vi "Build All.vi"() -> ()   [LabVIEW 2021]
uses:
  <vilib>/CIF Foundation/CIF LabVIEW Scripting/LV Scripting/Typedef/Version Increment.ctl
  <vilib>/CIF Foundation/CIF LabVIEW Scripting/LV Scripting/LV Scripting Utilities.lvlib
  <vilib>/AppBuilder/AB_API_Simple/NI_App_Builder_API.lvlib
  <vilib>/AppBuilder/AB_API_Simple/Build (path).vi
panel:
  in  "String":string
  in  "Changes":string
  in  "Version Increment":T1
  out "error out":errorcluster
  out "Description":string
  out "Version":T2
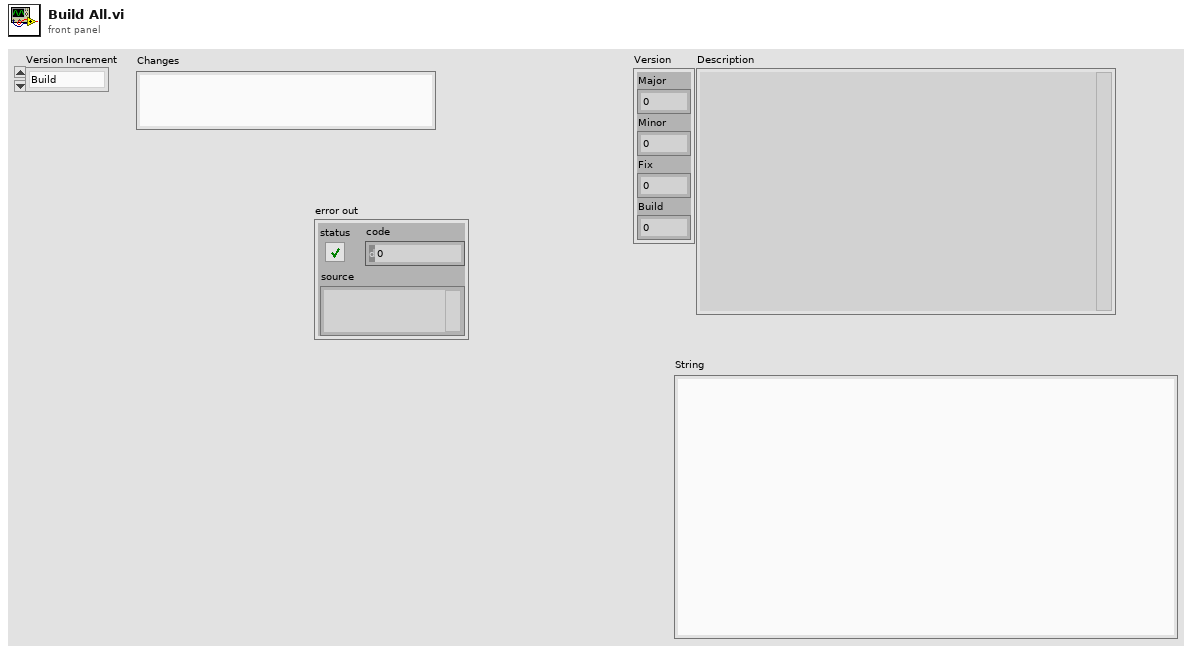
[diagram p1: front panel]
types:
  T1 = typedef "LV Scripting Utilities.lvlib/Version Increment.ctl" = enum16{"Build", "Fix", "Minor", "Major"}
  T2 = cluster{"Major":u16, "Minor":u16, "Fix":u16, "Build":u16}
  T3 = typedef "LV Scripting Utilities.lvlib/Target References.ctl" = cluster{"Target Reference":refnum<vi>, "VI References":refnum<vi>[], "Library References":refnum<vi>[], "Build References":refnum<vi>[]}
  T4 = typedef "LV Scripting Utilities.lvlib/BuildSpec Map.ctl" = map{string, refnum<vi>}
  T5 = typedef "LV Scripting Utilities.lvlib/Library Map.ctl" = map{string, refnum<vi>}
  T6 = typedef "Version.ctl" = cluster{"Major":u16, "Minor":u16, "Fix":u16, "Build":u16}
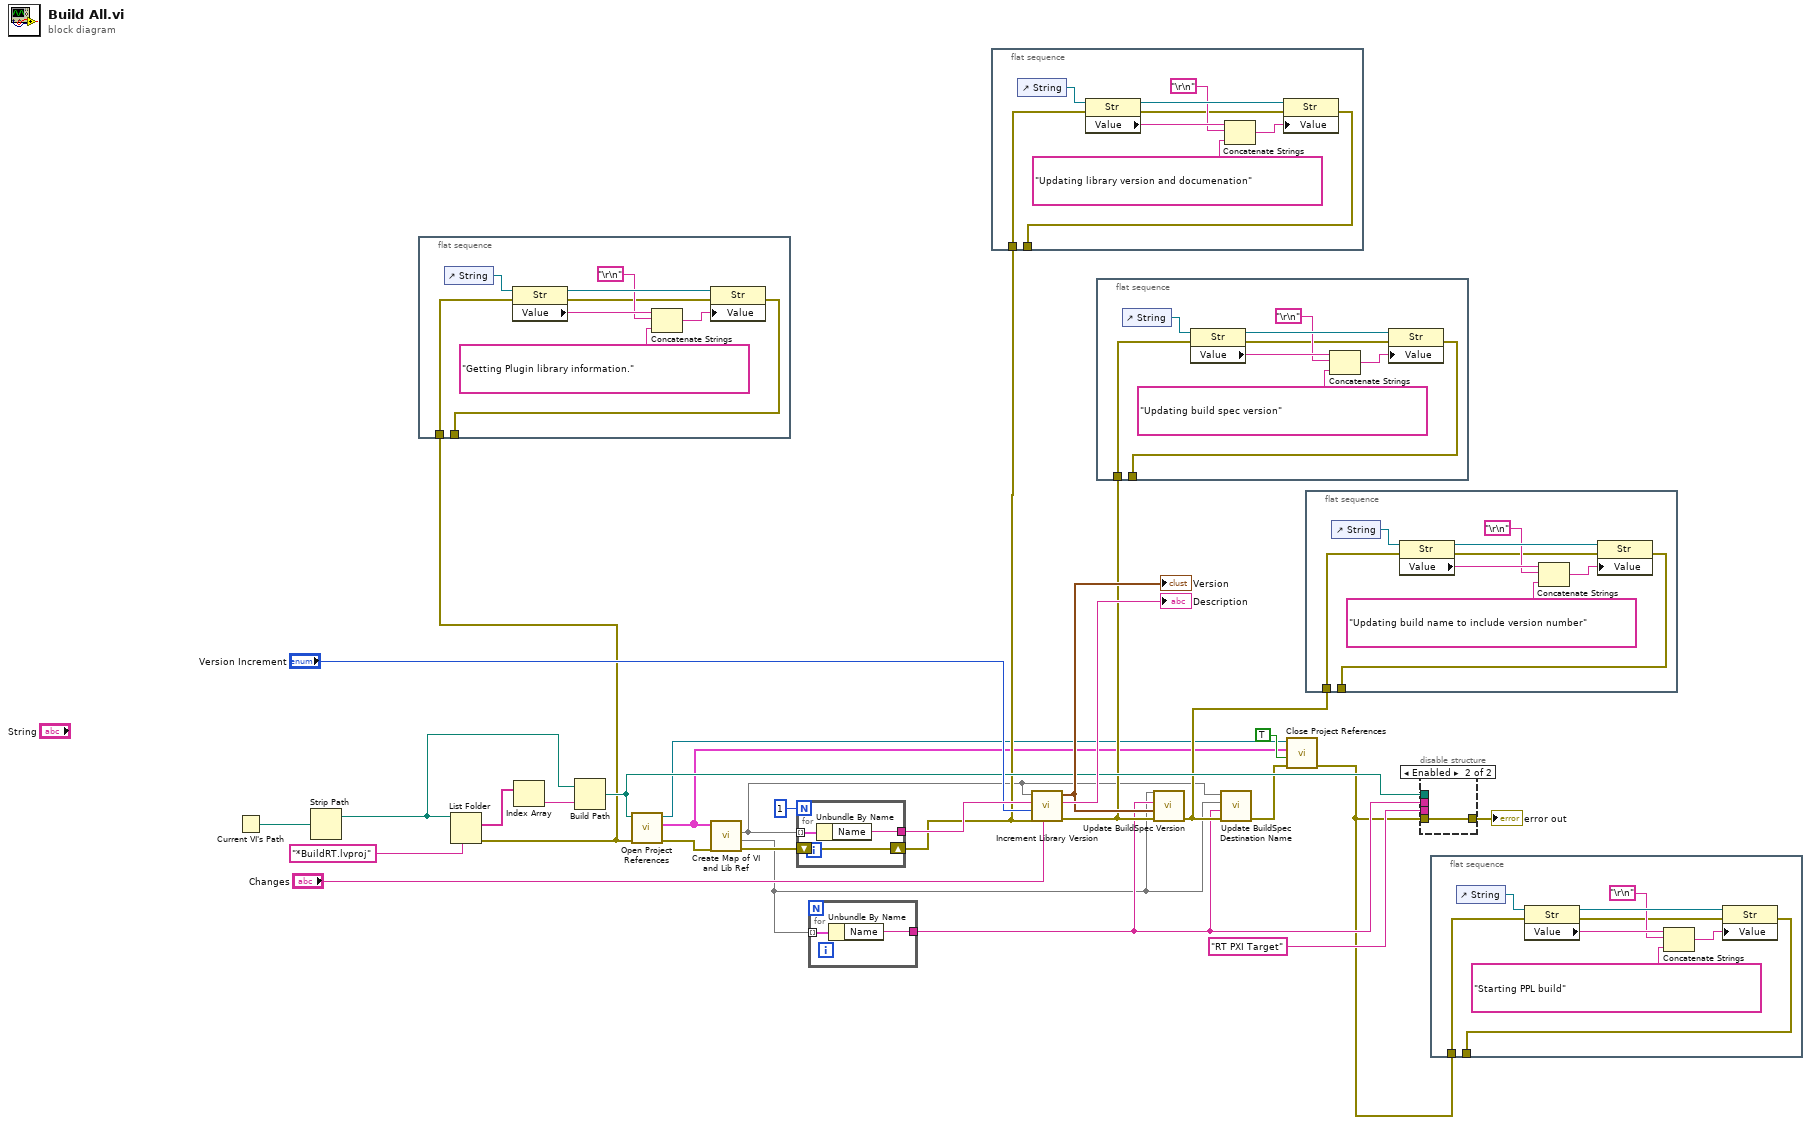
[diagram p0: block diagram]
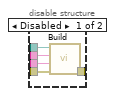
[diagram p2: hidden frame]
diagram:
  n1 = Current VI's Path() -> (path=w28:path)
  n2 = Strip Path(path=w28) -> (stripped path=w22:path)  [unwired: 1 out]
  n3 = flat-sequence {
    tunnel: w12 -> [w31]
    tunnel: [w29] -> _
    frame #0 {
      n4 = control-ref of="String"() -> (w37:refnum<vi>)
      n5 = property class="Str"(reference=w37, error in=w31) -> (reference out=w33:refnum<vi>, error out=w30:errorcluster, "Value"=w36:string)
      n6 = Concatenate Strings(w36, "\r\n", "Getting Plugin library information." ("Value")) -> (w34:string)
      n7 = property class="Str"(reference=w33, error in=w30, "Value"=w34) -> (error out=w29:errorcluster)  [unwired: 1 out]
    }
  }
  n8 = List Folder(path=w22, pattern="*BuildRT.lvproj") -> (filenames=w26:string[], error out=w12:errorcluster)  [unwired: 2 in, 2 out]
  n9 = Index Array(array=w26) -> (element=w23:string)  [unwired: 1 in]
  n10 = Build Path(base path=w22, name or relative path=w23) -> (appended path=w14:path)
  n11 = call <vilib>:"Open Project References.vi"("error in"=w12, "Project Path"=w14) -> ("error out"=w25:errorcluster, "VI, Library, and Build References"=w4:T3[], "Project Reference"=w5:refnum<vi>)  [unwired: 7 in]
  n12 = call <vilib>:"Create Map of VI and Lib Ref.vi"("error in"=w25, "VI, Library, and Build References"=w4) -> ("error out"=w20:errorcluster, "BuildSpec Map"=w7:T4, "Library Map"=w6:T5)  [unwired: 6 in, 1 out]
  n13 = for {
    N: 1 -> [_]
    tunnel: w6 -> [w40] mode=indexing
    tunnel: [w39] -> w19
    shift-right: [w38] -> w8
    shift-left: w20 -> [w38]
    n14 = Unbundle By Name(w40) -> ("Name"=w39:string)
  }
  n15 = for {
    tunnel: w7 -> [w42] mode=indexing
    tunnel: [w41] -> w9
    n16 = Unbundle By Name(w42) -> ("Name"=w41:string)
  }
  n17 = flat-sequence {
    tunnel: w8 -> [w45]
    tunnel: [w43] -> _
    frame #0 {
      n18 = control-ref of="String"() -> (w51:refnum<vi>)
      n19 = property class="Str"(reference=w51, error in=w45) -> (reference out=w47:refnum<vi>, error out=w44:errorcluster, "Value"=w50:string)
      n20 = Concatenate Strings(w50, "\r\n", "Updating library version and documenation" ("Value")) -> (w48:string)
      n21 = property class="Str"(reference=w47, error in=w44, "Value"=w48) -> (error out=w43:errorcluster)  [unwired: 1 out]
    }
  }
  n22 = call <vilib>:"Increment Library Version.vi"("Changes"="Changes", "error in (no error)"=w8, "Version Increment"="Version Increment", "Library Name"=w19, "Library Map"=w6) -> ("error out"=w11:errorcluster, "Description"=→"Description":string, "Version"=w15:T6)  [unwired: 4 in]
  "Version" <- w15
  n23 = flat-sequence {
    tunnel: w11 -> [w54]
    tunnel: [w52] -> _
    frame #0 {
      n24 = control-ref of="String"() -> (w60:refnum<vi>)
      n25 = property class="Str"(reference=w60, error in=w54) -> (reference out=w56:refnum<vi>, error out=w53:errorcluster, "Value"=w59:string)
      n26 = Concatenate Strings(w59, "\r\n", "Updating build spec version" ("Value")) -> (w57:string)
      n27 = property class="Str"(reference=w56, error in=w53, "Value"=w57) -> (error out=w52:errorcluster)  [unwired: 1 out]
    }
  }
  n28 = call <vilib>:"Update BuildSpec Version.vi"("error in (no error)"=w11, "New Version"=w15, "BuildSpec Name"=w9, "BuildSpec Map"=w7) -> ("error out"=w10:errorcluster)  [unwired: 7 in]
  n29 = call <vilib>:"Update BuildSpec Destination Name.vi"("error in (no error)"=w10, "BuildSpec Name"=w9, "BuildSpec Map"=w7, "Library Map"=w6) -> ("error out"=w3:errorcluster)  [unwired: 7 in]
  n30 = call <vilib>:"Close Project References.vi"("error in"=w3, "Save All"=TRUE, "VI, Library, and Build References"=w4, "Project Reference"=w5) -> ("error out"=w2:errorcluster)  [unwired: 7 in]
  n31 = flat-sequence {
    tunnel: w10 -> [w63]
    tunnel: [w61] -> _
    frame #0 {
      n32 = control-ref of="String"() -> (w69:refnum<vi>)
      n33 = property class="Str"(reference=w69, error in=w63) -> (reference out=w65:refnum<vi>, error out=w62:errorcluster, "Value"=w68:string)
      n34 = Concatenate Strings(w68, "\r\n", "Updating build name to include version number" ("Value")) -> (w66:string)
      n35 = property class="Str"(reference=w65, error in=w62, "Value"=w66) -> (error out=w61:errorcluster)  [unwired: 1 out]
    }
  }
  n36 = disable-structure shown="Enabled" {
    disable-tunnel: w14 -> [w74 _]
    disable-tunnel: "RT PXI Target" ("Name of target (My Computer)") -> [w73 _]
    disable-tunnel: w9 -> [w72 _]
    disable-tunnel: w2 -> [w71 w75]
    disable-tunnel: [w70 w75] -> w1
    frame Disabled {
      n37 = call-poly <vilib>:"Build.vi"("error in (no error)"=w71, "Name of target (My Computer)"=w73, "Name of build specification (if empty: build all)"=w72, "Path to project"=w74) -> ("error out"=w70:errorcluster)  [unwired: 6 in, 1 out]
    }
    frame Enabled {
    }
  }
  "error out" <- w1
  n38 = flat-sequence {
    tunnel: w2 -> [w78]
    tunnel: [w76] -> _
    frame #0 {
      n39 = control-ref of="String"() -> (w84:refnum<vi>)
      n40 = property class="Str"(reference=w84, error in=w78) -> (reference out=w80:refnum<vi>, error out=w77:errorcluster, "Value"=w83:string)
      n41 = Concatenate Strings(w83, "\r\n", "Starting PPL build" ("Value")) -> (w81:string)
      n42 = property class="Str"(reference=w80, error in=w77, "Value"=w81) -> (error out=w76:errorcluster)  [unwired: 1 out]
    }
  }
